vi "Initialize Sensors.vi"(11 "?":T1={"     Use ?\nOff       On"=[FALSE, TRUE, FALSE, TRUE], "Mode:"=FALSE, "WP Data"=0.0, "Hokuyo Port"="COM7", "Prop  Port"="COM6", "Compass Port"="", "GPS Port"=""}) -> (3 "?":T1={"     Use ?\nOff       On"=[FALSE, TRUE, FALSE, TRUE], "Mode:"=FALSE, "WP Data"=0.0, "Hokuyo Port"="COM7", "Prop  Port"="COM6", "Compass Port"="", "GPS Port"=""})   [LabVIEW 2014]
uses:
  Initialize-Standard.vi
  Hokuyo URG Series.lvlib
panel:
  in  "Checksum":bool
  in  "ID Query?":bool=TRUE
  in  "Protocol":u32(ring)=2 items=["Convert to Latest", "SCIP 1.1", "SCIP 2.0"]
  # "Initialize Sensors"
  # "Input:"
  # "Output:"
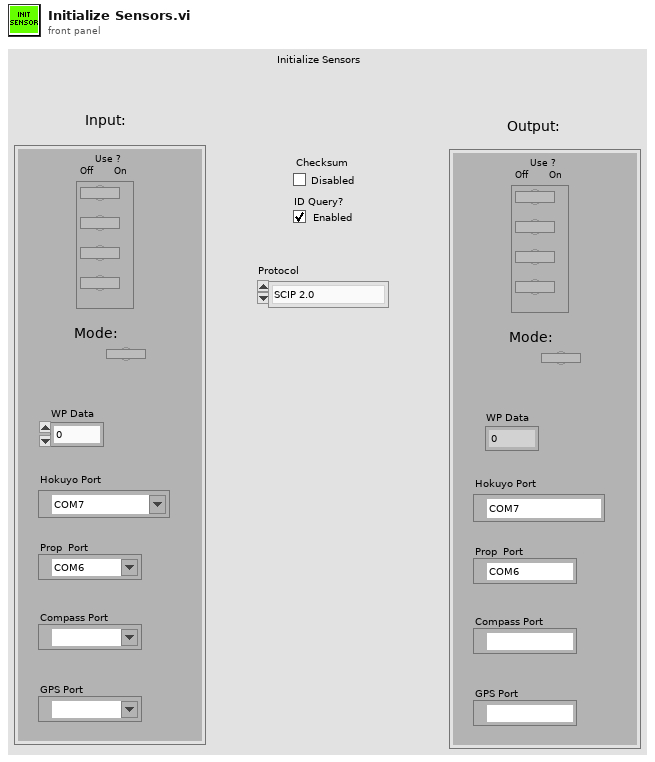
[diagram p1: front panel]
types:
  T1 = cluster{"     Use ?\nOff       On":bool[], "Mode:":bool, "WP Data":dbl, "Hokuyo Port":refnum<visa-resource-name>, "Prop  Port":refnum<visa-resource-name>, "Compass Port":refnum<visa-resource-name>, "GPS Port":refnum<visa-resource-name>}
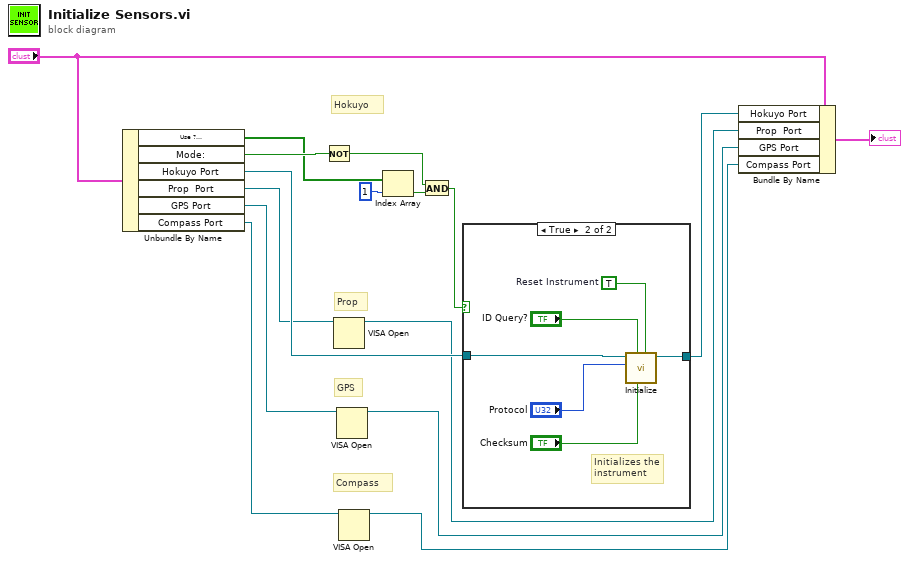
[diagram p0: block diagram]
diagram:
  # "Compass"
  # "GPS"
  # "Prop"
  # "Hokuyo"
  n1 = Unbundle By Name("?") -> ("Use ?\nOff       On"=w10:bool[], "Mode:"=w11:bool, "Hokuyo Port"=w13:refnum<visa-resource-name>, "Prop  Port"=w9:refnum<visa-resource-name>, "GPS Port"=w4:refnum<visa-resource-name>, "Compass Port"=w3:refnum<visa-resource-name>)
  n2 = Not(x=w11) -> (.not. x?=w14:bool)
  n3 = VISA Open(VISA resource name=w9) -> (VISA resource name=w7:refnum<visa-resource-name>)  [unwired: 4 in, 1 out]
  n4 = VISA Open(VISA resource name=w4) -> (VISA resource name=w2:refnum<visa-resource-name>)  [unwired: 4 in, 1 out]
  n5 = VISA Open(VISA resource name=w3) -> (VISA resource name=w1:refnum<visa-resource-name>)  [unwired: 4 in, 1 out]
  n6 = Index Array(array=w10, index=1) -> (element=w15:bool)
  n7 = And(x=w14, y=w15) -> (x .and. y?=w12:bool)
  n8 = case shown="True" w12 {
    tunnel: w13 -> [w17 w19]
    tunnel: [w17 w18] -> w8
    frame False {
    }
    frame True {
      w21 = TRUE  # Reset Instrument
      # "Initializes the instrument"
      n9 = call-poly "Initialize.vi"("Reset? (F: No)"=w21, "Checksum (Disabled)"="Checksum", "ID Query? (Enabled)"="ID Query?", "Protocol (2: SCIP 2.0)"="Protocol", "VISA resource name"=w19) -> ("VISA resource name out"=w18:refnum<visa-resource-name>)  [unwired: 5 in, 1 out]
    }
  }
  n10 = Bundle By Name(cluster="?", "Hokuyo Port"=w8, "Prop  Port"=w7, "GPS Port"=w2, "Compass Port"=w1) -> (→"?":T1)
